vi "Sensor Tests.vi"() -> ()   [LabVIEW 2012]
uses:
  Globals/Encoders Global.vi
  Globals/Potentiometers.vi
panel:
  out "Rate":dbl
  out "Act. Pot":dbl
  out "RR Pot":dbl
  out "RL Pot":dbl
  out "FR Pot":dbl
  out "FL Pot":dbl
  out "Shoot. Enc":dbl
  out "RR Enc":dbl
  out "RL Enc":dbl
  out "FR Enc":dbl
  out "FL Enc":dbl
  out "S3":bool
  out "S2":bool
  out "S1":bool
  out "IR":bool
  # "SWITCHBOX"
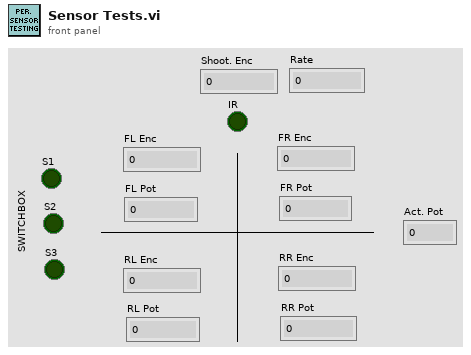
[diagram p1: front panel]
types:
  T1 = typedef "WPI_DigitalInputDevRef.ctl" = cluster{"DevStatus":errorcluster, "DIO Channel":T2, "Digital Module":T3}
  T2 = typedef "FPGA_DIOChannel.ctl" = enum8{"DIO 1", "DIO 2", "DIO 3", "DIO 4", "DIO 5", "DIO 6", "DIO 7", "DIO 8", "DIO 9", "DIO 10", "DIO 11", "DIO 12", "DIO 13", "DIO 14", "Invalid"}
  T3 = typedef "FPGA_TypedefDigitalModule.ctl" = enum16{"Digital Module 1", "Digital Module 2"}
  T4 = typedef "WPI_AnalogChannelDevRef.ctl" = cluster{"DevStatus":errorcluster, "Analog Module":T5, "Analog Channel":T6}
  T5 = typedef "FPGA_TypedefAnalogModule.ctl" = enum16{"Analog Module 1", "Analog Module 2"}
  T6 = typedef "FPGA_AIChannel.ctl" = enum8{"AI 1", "AI 2", "AI 3", "AI 4", "AI 5", "AI 6", "AI 7", "AI 8", "Invalid"}
  T7 = cluster{"Front Left":T4, "Front Right":T4, "Rear Left":T4, "Rear Right":T4, "Actuator":T4}
  T8 = typedef "WPI_EncoderDevRef.ctl" = cluster{"DevStatus":errorcluster, "EncoderIndex":T9, "CounterIndex":T10, "DistancePerCount":dbl, "Decoding Type":T11}
  T9 = typedef "FPGA_EncoderIdx.ctl" = enum8{"Enc 0", "Enc 1", "Enc 2", "Enc 3", "Invalid"}
  T10 = typedef "FPGA_CounterCtrSystemIndex.ctl" = enum8{"Ctr 0", "Ctr 1", "Ctr 2", "Ctr 3", "Ctr 4", "Ctr 5", "Ctr 6", "Ctr 7", "Invalid"}
  T11 = typedef "WPI_EncoderType.ctl" = enum16{"1x", "2x", "4x"}
  T12 = cluster{"Front Left":T8, "Front Right":T8, "Rear Left":T8, "Rear Right":T8, "Shooter":T8}
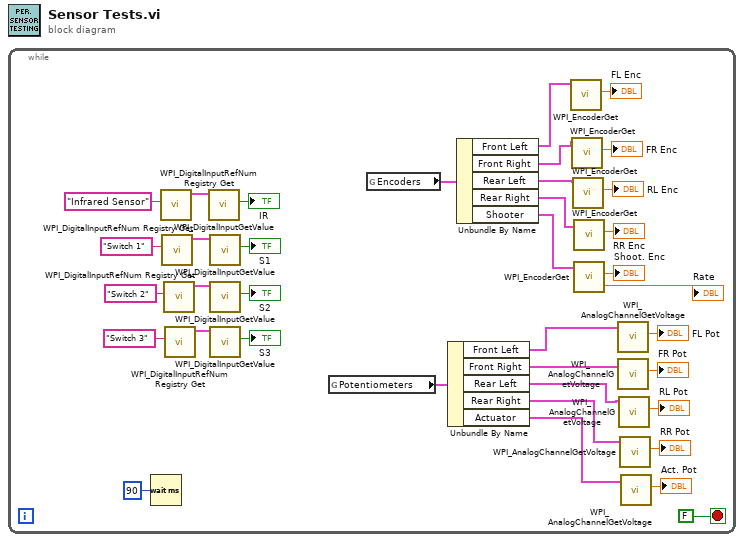
[diagram p0: block diagram]
diagram:
  n1 = while {
    stop <- FALSE stop-if-true
    n2 = Wait (ms)(milliseconds to wait=u32 90) -> ()  [unwired: 1 out]
    n3 = call <vilib>:"WPI_DigitalInputRefNum Registry Get.vi"("refnum name"="Infrared Sensor") -> ("DigitalInputDevRef"=w33:T1)  [unwired: 9 in, 1 out]
    n4 = call <vilib>:"WPI_DigitalInputRefNum Registry Get.vi"("refnum name"="Switch 1") -> ("DigitalInputDevRef"=w32:T1)  [unwired: 9 in, 1 out]
    n5 = call <vilib>:"WPI_DigitalInputRefNum Registry Get.vi"("refnum name"="Switch 2") -> ("DigitalInputDevRef"=w31:T1)  [unwired: 9 in, 1 out]
    n6 = call <vilib>:"WPI_DigitalInputRefNum Registry Get.vi"("refnum name"="Switch 3") -> ("DigitalInputDevRef"=w30:T1)  [unwired: 9 in, 1 out]
    n7 = call <vilib>:"WPI_DigitalInputGetValue.vi"("DigitalInputDevRef"=w33) -> ("Value"=→"IR":bool)  [unwired: 8 in, 2 out]
    n8 = call <vilib>:"WPI_DigitalInputGetValue.vi"("DigitalInputDevRef"=w32) -> ("Value"=→"S1":bool)  [unwired: 8 in, 2 out]
    n9 = call <vilib>:"WPI_DigitalInputGetValue.vi"("DigitalInputDevRef"=w31) -> ("Value"=→"S2":bool)  [unwired: 8 in, 2 out]
    n10 = call <vilib>:"WPI_DigitalInputGetValue.vi"("DigitalInputDevRef"=w30) -> ("Value"=→"S3":bool)  [unwired: 8 in, 2 out]
    n11 = global read "Potentiometers.vi" "Potentiometers"() -> (w14:T7)
    n12 = global read "Encoders Global.vi" "Encoders"() -> (w25:T12)
    n13 = Unbundle By Name(w14) -> ("Front Left"=w13:T4, "Front Right"=w12:T4, "Rear Left"=w11:T4, "Rear Right"=w10:T4, "Actuator"=w9:T4)
    n14 = Unbundle By Name(w25) -> ("Front Left"=w24:T8, "Front Right"=w23:T8, "Rear Left"=w22:T8, "Rear Right"=w21:T8, "Shooter"=w20:T8)
    n15 = call <vilib>:"WPI_EncoderGet.vi"("EncoderDevRef"=w24) -> ("Distance"=→"FL Enc":dbl)  [unwired: 5 in, 5 out]
    n16 = call <vilib>:"WPI_EncoderGet.vi"("EncoderDevRef"=w23) -> ("Distance"=→"FR Enc":dbl)  [unwired: 5 in, 5 out]
    n17 = call <vilib>:"WPI_EncoderGet.vi"("EncoderDevRef"=w22) -> ("Distance"=→"RL Enc":dbl)  [unwired: 5 in, 5 out]
    n18 = call <vilib>:"WPI_EncoderGet.vi"("EncoderDevRef"=w21) -> ("Distance"=→"RR Enc":dbl)  [unwired: 5 in, 5 out]
    n19 = call <vilib>:"WPI_EncoderGet.vi"("EncoderDevRef"=w20) -> ("Distance"=→"Shoot. Enc":dbl, "Rate"=→"Rate":dbl)  [unwired: 5 in, 4 out]
    n20 = call <vilib>:"WPI_AnalogChannelGetVoltage.vi"("AIDeviceRef"=w13) -> ("Voltage"=→"FL Pot":dbl)  [unwired: 8 in, 2 out]
    n21 = call <vilib>:"WPI_AnalogChannelGetVoltage.vi"("AIDeviceRef"=w12) -> ("Voltage"=→"FR Pot":dbl)  [unwired: 8 in, 2 out]
    n22 = call <vilib>:"WPI_AnalogChannelGetVoltage.vi"("AIDeviceRef"=w11) -> ("Voltage"=→"RL Pot":dbl)  [unwired: 8 in, 2 out]
    n23 = call <vilib>:"WPI_AnalogChannelGetVoltage.vi"("AIDeviceRef"=w10) -> ("Voltage"=→"RR Pot":dbl)  [unwired: 8 in, 2 out]
    n24 = call <vilib>:"WPI_AnalogChannelGetVoltage.vi"("AIDeviceRef"=w9) -> ("Voltage"=→"Act. Pot":dbl)  [unwired: 8 in, 2 out]
  }
